vi "rsp_Connection Notify.vi"(8 "error in":errorcluster, 9 "Data in":T1={"Connected?"=FALSE, "DC_UID"="", "Message Priority"=enum."Normal", "IP Address"=""}, 11 "DS TCP Server in":refnum<class "DS TCP Server.lvclass">) -> (0 "error out":errorcluster, 3 "dup DS TCP Server out":refnum<class "DS TCP Server.lvclass">)   [LabVIEW 2017, in "DS TCP Server.lvlib" / "DS TCP Server.lvclass"]
doc: "This VI sends a <b>Public API Response</b> message to a registered MHL case of the Caller of the Worker that owns this VI.\n---"
uses:
  DS TCP Server.lvclass
  C:/Program Files (x86)/National Instruments/LabVIEW 2017/vi.lib/addons/_Workers/Library/Classes/Worker/Worker.lvclass
  rsp_Connection Notify.ctl
  Common VIs/DC_UID.ctl
  <vilib>/addons/_Workers/Library/Classes/Message/Priority.ctl
  DS TCP Server.lvclass/DS TCP Server.ctl
  <vilib>/addons/_Workers/Library/Classes/Worker/Worker.lvclass/Worker.ctl
  <vilib>/Utility/error.llb/Error Cluster From Error Code.vi
  <vilib>/addons/_Workers/Library/Classes/Message/Enqueue Message to Queue.vi
  <vilib>/ErrorRing/Error Ring.xnode
  <vilib>/addons/_Workers/Library/Classes/Message/Message.lvclass
  <vilib>/addons/_Workers/Library/Classes/Worker/Worker.lvclass
  C:/Program Files (x86)/National Instruments/LabVIEW 2017/vi.lib/addons/_Workers/Library/Classes/Workers Object/Workers Object.lvclass
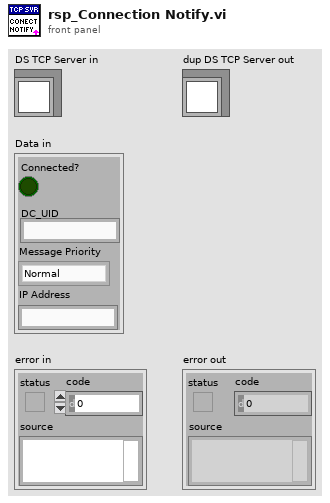
[diagram p1: front panel]
types:
  T1 = typedef "DS TCP Server.lvlib/DS TCP Server.lvclass/rsp_Connection Notify.ctl" = cluster{"Connected?":bool, "DC_UID":T2, "Message Priority":T3, "IP Address":string}
  T2 = typedef "DC_UID.ctl" = string
  T3 = typedef "Workers.lvlib/Message.lvclass/Priority.ctl" = enum16{"Low", "Normal", "High"}
  T4 = typedef "Workers.lvlib/Case Label.ctl" = string
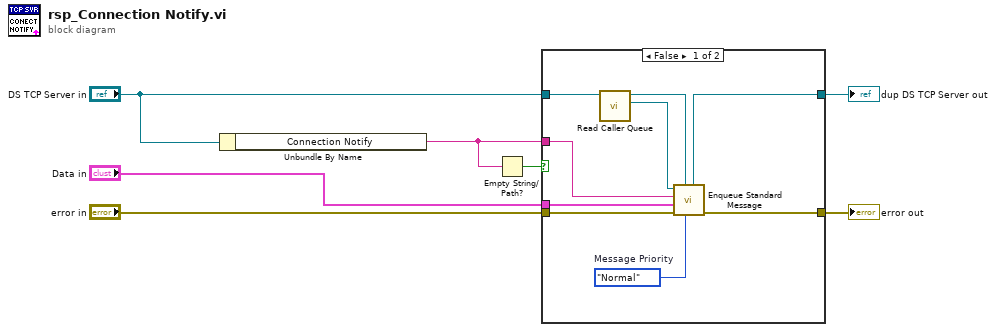
[diagram p0: block diagram]
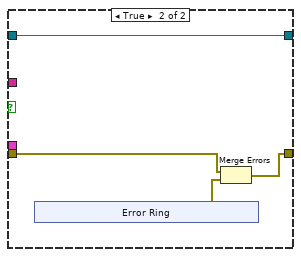
[diagram p2: hidden frame]
diagram:
  n1 = Unbundle By Name("DS TCP Server in") -> ("Connection Notify"=w2:T4)
  n2 = Empty String/Path?(string/path=w2) -> (empty?=w3:bool)
  n3 = case shown="False" w3 {
    tunnel: "error in" -> [w10 w18]
    tunnel: [w16 w17] -> w6
    tunnel: "Data in" -> [w14 _]
    tunnel: [w13 w20] -> w4
    tunnel: "DS TCP Server in" -> [w11 w20]
    tunnel: w2 -> [w12 _]
    frame False {
      w15 = Priority."Normal"  # Message Priority
      n4 = call <vilib>:"Read Caller Queue.vi"("Worker_"=w11) -> ("Message Queue out"=w8:refnum<class "Message Queue.lvclass">, "dup Worker_out"=w9:refnum<class "DS TCP Server.lvclass">)  [unwired: 9 in]
      n5 = call-poly <vilib>:"Enqueue Standard Message.vi"("Priority (Normal)"=w15, "Worker"=w9, "error in"=w10, "Data"=w14, "Case Label"=w12, "Message Queue"=w8) -> ("error out"=w16:errorcluster, "dup Worker out"=w13:refnum<class "DS TCP Server.lvclass">)  [unwired: 3 in, 1 out]
    }
    frame True {
      n6 = xnode "Error Ring"() -> ("error out"=w19:errorcluster)
      n7 = Merge Errors(w18, w19) -> (w17:errorcluster)
    }
  }
  "error out" <- w6
  "dup DS TCP Server out" <- w4
